vi "Runner.ItemsToPathArray.vi"(10 "Project Items":refnum<vi>[](array[refnum])) -> (1 "Paths":path[](array[path]))   [LabVIEW 2013, in "Caraya.lvlib" / "Test Runner.lvclass"]
uses:
  Test Runner.lvclass
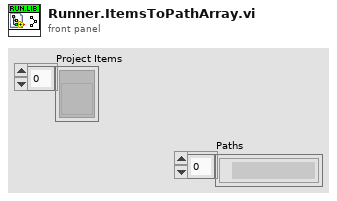
[diagram p1: front panel]
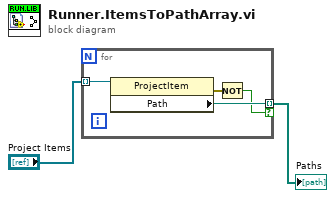
[diagram p0: block diagram]
diagram:
  n1 = for {
    tunnel: "Project Items" -> [w6] mode=indexing
    tunnel: [w5] -> w2 mode=indexing if=w3
    n2 = property class="ProjectItem"(reference=w6) -> (error out=w4:errorcluster, "Path"=w5:path)  [unwired: 1 in, 1 out]
    n3 = Not(x=w4) -> (.not. x?=w3:bool)
  }
  "Paths" <- w2
